vi "compressor_getdetailedenablstate.vi"(0 "CompressorDevRef":T1, 11 "error in (no error)":errorcluster) -> (4 "CompressorDevRef":T1, 6 "Enabled":bool, 10 "Compressor Running":bool, 12 "On/Off":bool, 13 "Charging":bool, 14 "Full":bool, 15 "error out":errorcluster)   [LabVIEW 2014]
doc: "Returns the enable/start state of the compressor and the on/off state of the compressor relay.\n\nThis software is licensed. Open the labview\\readme\\WPI Robotics Library Open Source License.txt file for more information."
uses:
  <vilib>/Rock Robotics/WPI/Compressor/WPI_CompressorDevRef.ctl
panel:
  # "Modified Compresser VI to Output More Information"
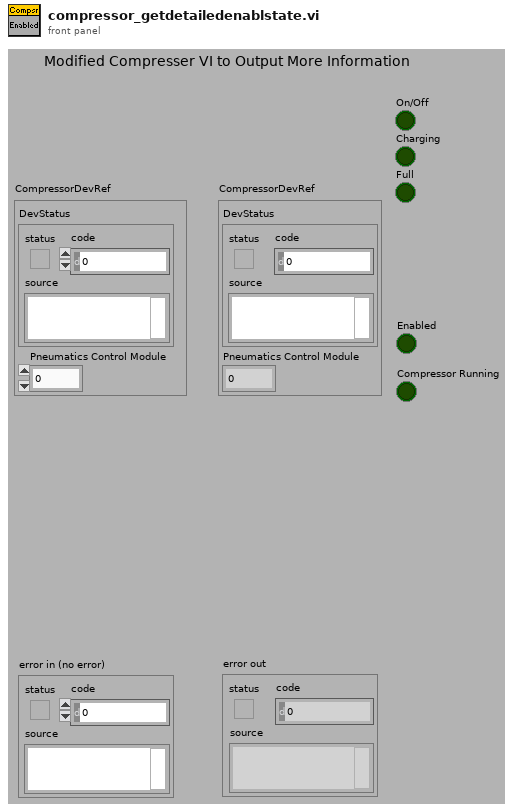
[diagram p1: front panel]
types:
  T1 = typedef "WPI_CompressorDevRef.ctl" = cluster{"DevStatus":errorcluster, "Pneumatics Control Module":u8}
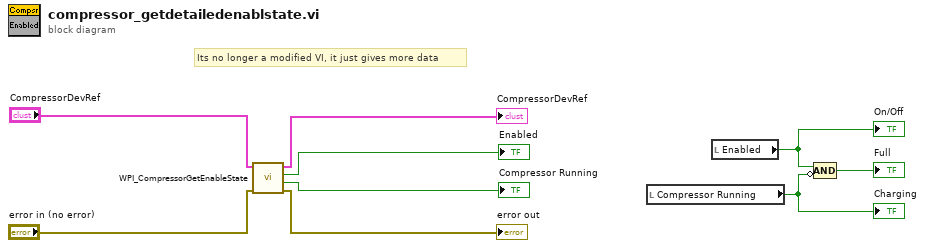
[diagram p0: block diagram]
diagram:
  # "Its no longer a modified VI, it just gives more data"
  n1 = call <vilib>:"WPI_CompressorGetEnableState.vi"("error in (no error)"="error in (no error)", "CompressorDevRef"="CompressorDevRef") -> ("error out"=→"error out":errorcluster, "Compressor Running"=→"Compressor Running":bool, "Enabled"=→"Enabled":bool, "CompressorDevRef"=→"CompressorDevRef":T1)  [unwired: 6 in]
  n2 = local read "Compressor Running"() -> (w7:bool)
  "Charging" <- w7
  n3 = local read "Enabled"() -> (w8:bool)
  "On/Off" <- w8
  n4 = Compound Arithmetic op=AND(w8, invert w7) -> (→"Full":bool)
